vi "Simulation 01.vi"() -> ()   [LabVIEW 2014]
uses:
  <vilib>/Motion/BlockNode/FB.NIMotion.xnode
  <vilib>/Motion/Express/_s/nimc.fb.straightLineMove.startStraightLineMove.axis.modeAbsolute.0.vi
panel:
  out "done 2":bool
  in  "acceleration 2":dbl=90.0
  in  "velocity 2":dbl=360.0
  in  "position 2":dbl=3600.0
  in  "execute 2":bool
  in  "Stop Button":bool
  out "done":bool
  in  "acceleration":dbl=90.0
  in  "velocity":dbl=360.0
  in  "position":dbl=7200.0
  in  "execute":bool
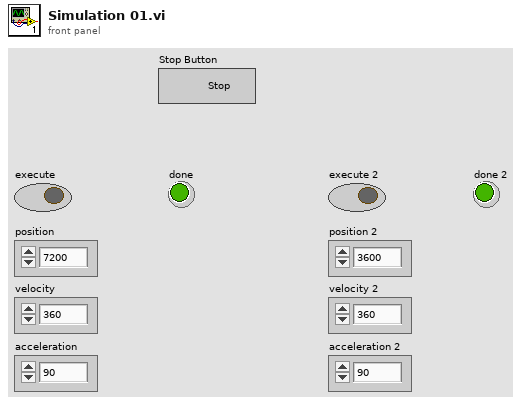
[diagram p1: front panel]
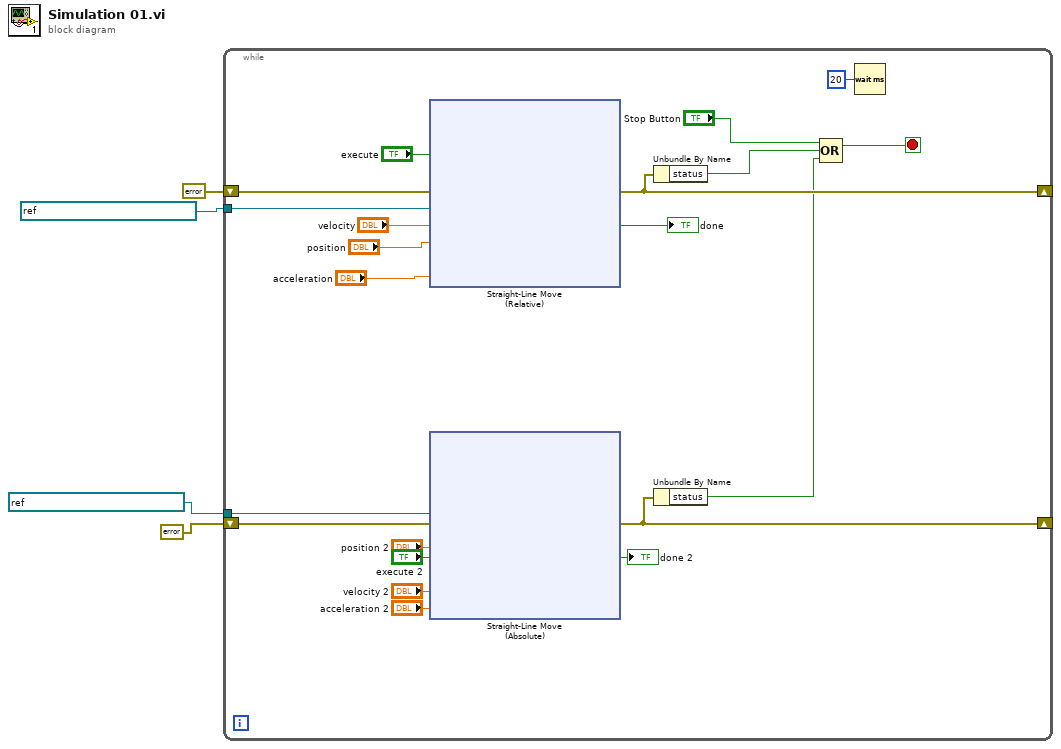
[diagram p0: block diagram]
diagram:
  n1 = while {
    shift-right: [w17] -> _
    shift-left: errorcluster {"status"=FALSE, "code"=0, "source"=""} ("error in") -> [w19]
    tunnel: refnum<k21> "nism://My Computer/Axis 1" ("resource") -> [w18]
    tunnel: refnum<k21> "nism://My Computer/Axis 2" ("resource") -> [w8]
    shift-right: [w6] -> _
    shift-left: errorcluster {"status"=FALSE, "code"=0, "source"=""} ("error in") -> [w7]
    stop <- w14 stop-if-true
    n2 = xnode "Straight-Line Move\n(Relative)"("error in"=w19, "resource"=w18, "execute"="execute", "position"="position", "velocity"="velocity", "acceleration"="acceleration") -> ("error out"=w17:errorcluster, "done"=→"done":bool)  [unwired: 1 out]
    n3 = xnode "Straight-Line Move\n(Absolute)"("error in"=w7, "resource"=w8, "execute"="execute 2", "position"="position 2", "velocity"="velocity 2", "acceleration"="acceleration 2") -> ("error out"=w6:errorcluster, "done"=→"done 2":bool)  [unwired: 1 out]
    n4 = Unbundle By Name(w17) -> ("status"=w15:bool)
    n5 = Unbundle By Name(w6) -> ("status"=w5:bool)
    n6 = Compound Arithmetic op=OR("Stop Button", w15, w5) -> (w14:bool)
    n7 = Wait (ms)(milliseconds to wait=u32 20) -> ()  [unwired: 1 out]
  }
